vi "testarray.vi"() -> ()   [LabVIEW 2017]
panel:
  out "Array 2":dbl[](array[numeric])
  in  "Array":dbl[](array[numeric])
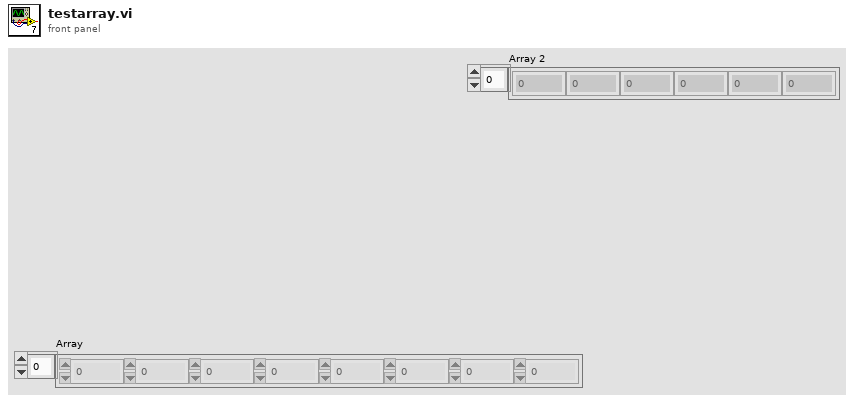
[diagram p1: front panel]
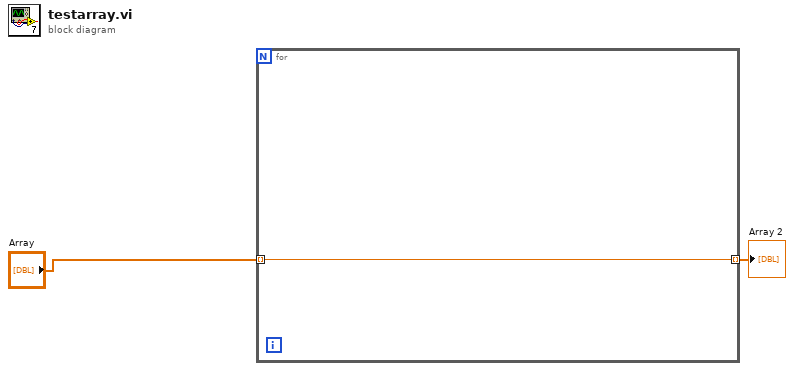
[diagram p0: block diagram]
diagram:
  n1 = for {
    tunnel: [w3] -> w1 mode=indexing
    tunnel: "Array" -> [w3] mode=indexing
  }
  "Array 2" <- w1
